vi "rotate 2D array V0.vi"(9 "rotate y":i32=1, 10 "rotate x":i32, 11 "array in":cdb[][](array[numeric])=[[0.0+0.0i, 1.0+0.0i, 2.0+0.0i, 3.0+0.0i], [4.0+0.0i, 0.0+0.0i, 0.0+0.0i, 0.0+0.0i], [8.0+0.0i, 0.0+0.0i, 0.0+0.0i, 0.0+0.0i], [13.0+0.0i, 0.0+0.0i, 99.0+0.0i, 0.0+0.0i]]) -> (3 "array out":cdb[][](array[numeric])=[[13.0+0.0i, 0.0+0.0i, 99.0+0.0i, 0.0+0.0i], [0.0+0.0i, 1.0+0.0i, 2.0+0.0i, 3.0+0.0i], [4.0+0.0i, 0.0+0.0i, 0.0+0.0i, 0.0+0.0i], [8.0+0.0i, 0.0+0.0i, 0.0+0.0i, 0.0+0.0i]])   [LabVIEW 2010]
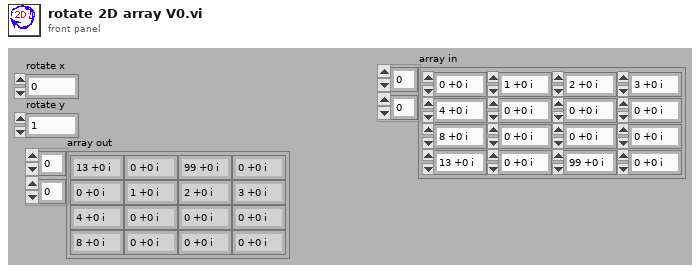
[diagram p1: front panel]
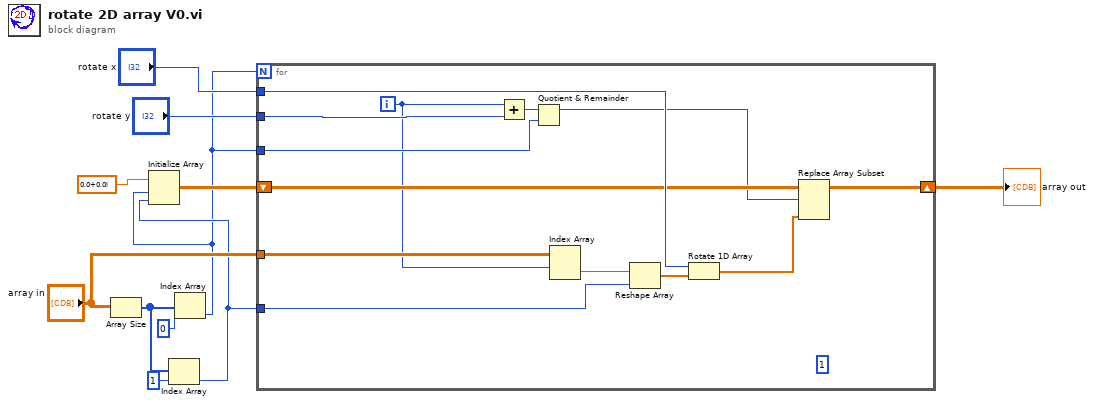
[diagram p0: block diagram]
diagram:
  n1 = Array Size(array="array in") -> (size(s)=w8:i32[])
  n2 = Index Array(array=w8, index=1) -> (element=w4:i32)
  n3 = Index Array(array=w8, index=0) -> (element=w1:i32)
  n4 = Initialize Array(cdb 0.0+0.0i ("element"), w1, w4) -> (w7:cdb[][])
  n5 = for {
    N: w1 -> [_]
    tunnel: w1 -> [w24]
    shift-right: [w17] -> w2
    shift-left: w7 -> [w19]
    tunnel: "rotate y" -> [w22]
    tunnel: "array in" -> [w15]
    tunnel: w4 -> [w16]
    tunnel: "rotate x" -> [w20]
    i -> [w14]
    (unwired) 1 ("dimension size")
    n6 = Add(x=w14, y=w22) -> (x+y=w23:i32)
    n7 = Quotient & Remainder(x=w23, y=w24) -> (x-y*floor(x/y)=w18:i32)  [unwired: 1 out]
    n8 = Index Array(array=w15, index (row)=w14) -> (element=w13:cdb[])  [unwired: 1 in]
    n9 = Reshape Array(w13, w16) -> (w21:cdb[])
    n10 = Rotate 1D Array(1:w21, 2:w20) -> (0:w12:cdb[])
    n11 = Replace Array Subset(array=w19, new element=w12, index (row)=w18) -> (w17:cdb[][])  [unwired: 1 in]
  }
  "array out" <- w2
